vi "InstrumentSelection.vi"(8 "error in (no error)":errorcluster, 9 "Verify GPIB address":bool, 10 "Instrument type":T1(ring), 11 "Instrument name IN":string(combo)) -> (0 "error out":errorcluster, 1 "Instrument name OUT":string, 2 "LCR":refnum<class "LCRControl.lvclass">, 3 "Supply":refnum<class "SupplyControl.lvclass">, 4 "Switching":refnum<class "Switching.lvclass">, 5 "Multimeter":refnum<class "MultimeterControl.lvclass">)   [LabVIEW 2019, in "InstrControl.lvclass"]
uses:
  InstrControl.lvclass
  SupplyControl/SupplyControl.lvclass
  C:/Users/probe/Desktop/TRIUMF-Dark-Box/InstrControl/InstrControl.lvclass
  LCRControl/LCRControl.lvclass
  MultimeterControl/MultimeterControl.lvclass
  Switching/Switching.lvclass
  SupplyControl/Keithley 2410/KE2410.lvclass
  C:/Users/probe/Desktop/TRIUMF-Dark-Box/InstrControl/SupplyControl/SupplyControl.lvclass
  SupplyControl/Keithley 6517/KE6517.lvclass
  SupplyControl/Keithley 487/KE487.lvclass
  SupplyControl/Keithley 236 & 237/KE236.lvclass
  LCRControl/WK6440B/WK6440B.lvclass
  C:/Users/probe/Desktop/TRIUMF-Dark-Box/InstrControl/LCRControl/LCRControl.lvclass
  LCRControl/WK6425/WK6425.lvclass
  MultimeterControl/Keithley 2000/KE2000.lvclass
  C:/Users/probe/Desktop/TRIUMF-Dark-Box/InstrControl/MultimeterControl/MultimeterControl.lvclass
  Switching/Pickering/Pickering.lvclass
  C:/Users/probe/Desktop/TRIUMF-Dark-Box/InstrControl/Switching/Switching.lvclass
  InstrumentSetup.vi
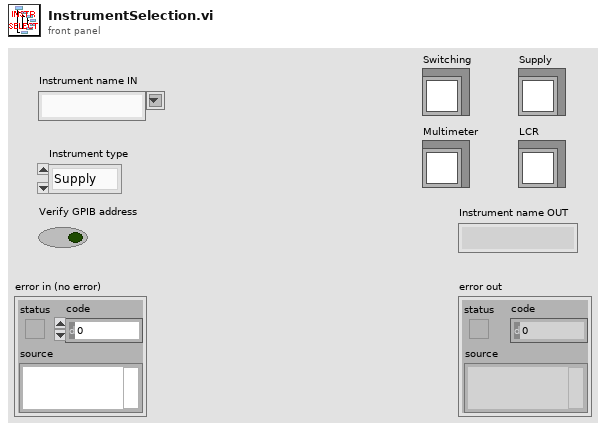
[diagram p1: front panel]
types:
  T1 = enum16{"Supply", "LCR", "Multimeter", "Switching"}
  T2 = cluster{"KE 2410":cluster{"Instrument name":string, "GPIB address":string, "Instrument type":u16}, "KE 6517":cluster{"Instrument name":string, "GPIB address":string, "Instrument type":u16}, "KE 487":cluster{"Instrument name":string, "GPIB address":string, "Instrument type":u16}, "KE 236":cluster{"Instrument name":string, "GPIB address":string, "Instrument type":u16}, "KE 487_2":cluster{"Instrument name":string, "GPIB address":string, "Instrument type":u16}, "WK 6440B":cluster{"Instrument name":string, "GPIB address":string, "Instrument type":u16}, "WK 6425":cluster{"Instrument name":string, "GPIB address":string, "Instrument type":u16}, "Pickering Matrix":cluster{"Instrument name":string, "GPIB address":string, "Instrument type":u16}, "KE 2000":cluster{"Instrument name":string, "GPIB address":string, "Instrument type":u16}, "KE3706A Switching":cluster{"Instrument name":string, "GPIB address":string, "Instrument type":u16}}
  T3 = cluster{"Current Limit":sgl, "KE2410":refnum<class "KE2410.lvclass">}
  T4 = cluster{"Current Limit":u16, "KE6517":refnum<class "KE6517.lvclass">}
  T5 = cluster{"Compliance":u16, "Range:":u16, "KE487":refnum<class "KE487.lvclass">}
  T6 = cluster{"current \ncompliance level":dbl, "compliance/\nmeasurement range (auto:0)":u16, "KE236":refnum<class "KE236.lvclass">}
  T7 = cluster{"RC Configuration":u16, "AC amplitude [V]":dbl, "AC frequency [Hz]":i32, "WK6440B":refnum<class "WK6440B.lvclass">}
  T8 = cluster{"RC Configuration":u16, "AC amplitude [V]":dbl, "AC frequency [Hz]":i32, "WK6425":refnum<class "WK6425.lvclass">}
  T9 = cluster{"Range":u16, "Range Value":dbl, "Function":u16, "KE2000":refnum<class "KE2000.lvclass">}
  T10 = cluster{"Matrix address":string, "Mux1 address":string, "Mux2 address":string, "Matrix used?":bool, "Pickering":refnum<class "Pickering.lvclass">, "Matrix X Channels":cluster{"Bias Supply / SMU LO":i32, "Bias Supply / SMU HI":i32, "CV Box LO":i32, "CV Box HI":i32, "CV Box LO IN":i32, "CV Box HI IN":i32, "Volt meter LO":i32, "Volt meter HI":i32, "Mux1 C1":i32, "Mux1 C2":i32, "Mux2 C1":i32, "Mux2 C2":i32}}
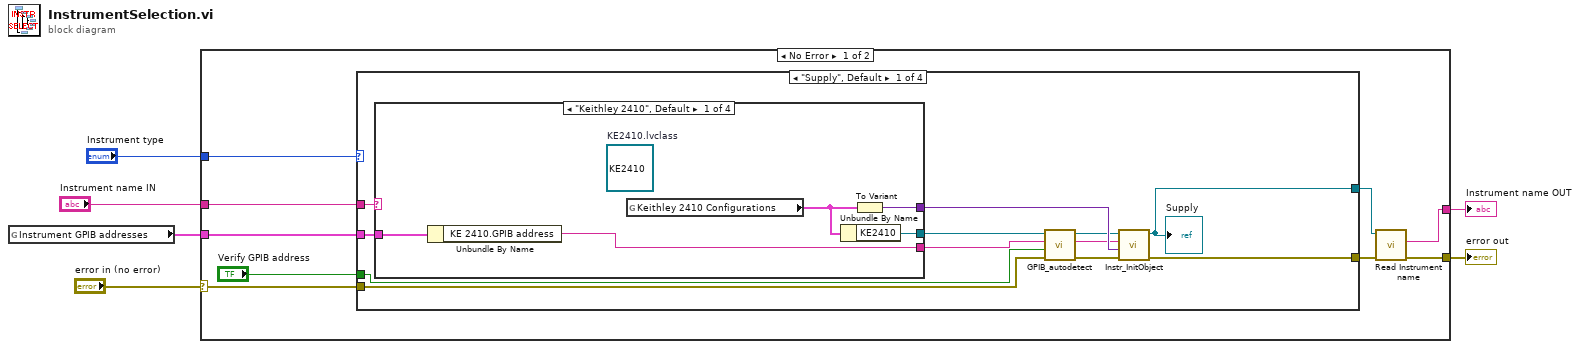
[diagram p0: block diagram]
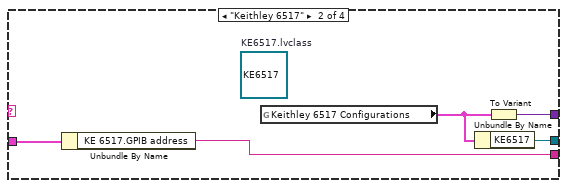
[diagram p2: hidden frame]
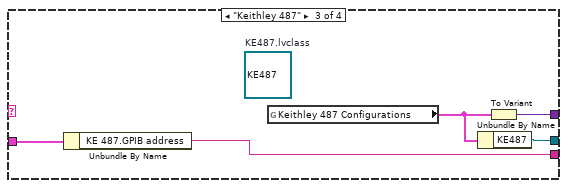
[diagram p3: hidden frame]
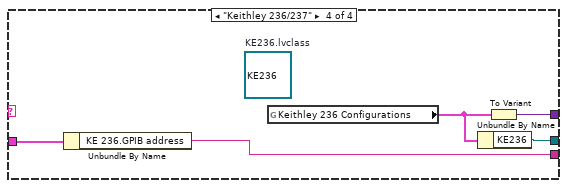
[diagram p4: hidden frame]
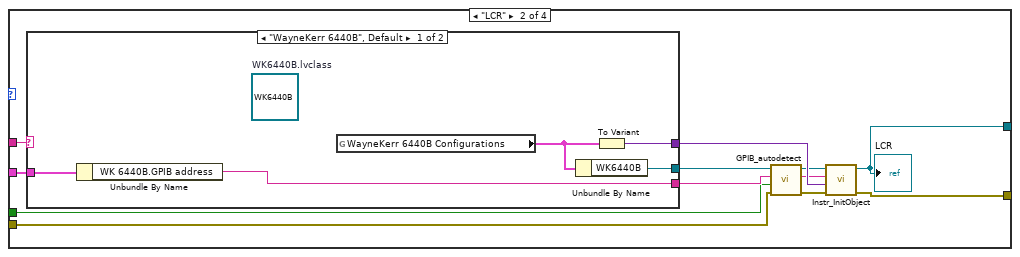
[diagram p5: hidden frame]
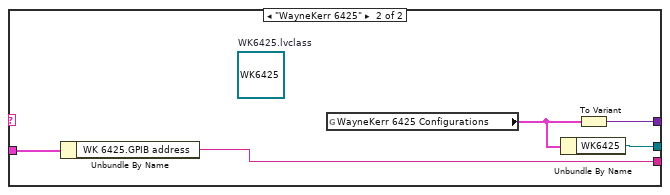
[diagram p6: hidden frame]
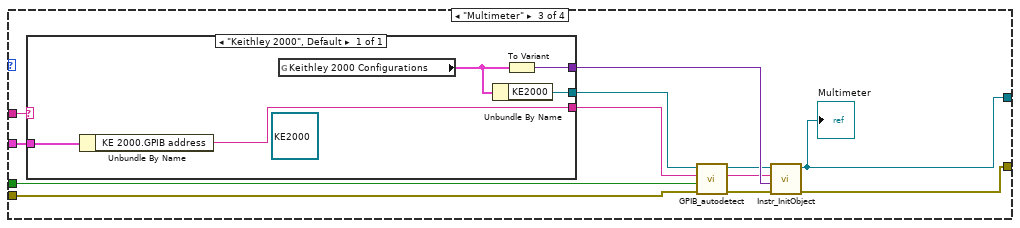
[diagram p7: hidden frame]
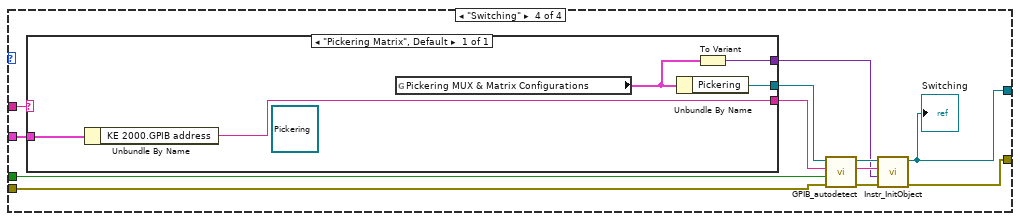
[diagram p8: hidden frame]
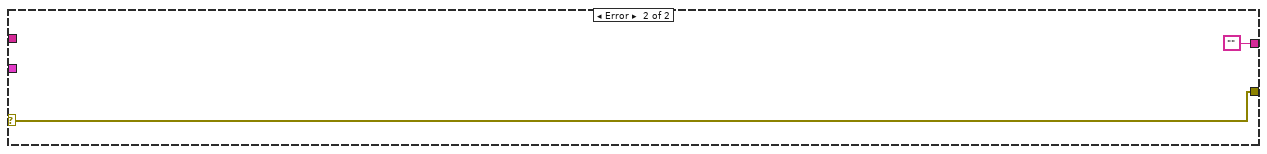
[diagram p9: hidden frame]
diagram:
  n1 = global read "InstrumentSetup.vi" "Instrument GPIB addresses"() -> (w1:T2)
  n2 = case shown="No Error" "error in (no error)" {
    selector: "error in (no error)" -> [w13 w105]
    tunnel: [w14 w105] -> w5
    tunnel: [w15 ""] -> w4
    tunnel: "Instrument type" -> [w10 _]
    tunnel: "Instrument name IN" -> [w9 _]
    tunnel: w1 -> [w8 _]
    frame No Error {
      n3 = case shown="\"Supply\", Default" w10 {
        tunnel: w9 -> [w27 w59 w81 w89]
        tunnel: [w26 w57 w79 w97] -> w12
        tunnel: w13 -> [w18 w54 w71 w91]
        tunnel: [w25 w58 w80 w98] -> w11
        tunnel: w8 -> [w24 w56 w78 w95]
        tunnel: "Verify GPIB address" -> [w17 w48 w76 w90]
        frame "Supply", Default {
          n4 = case shown="\"Keithley 2410\", Default" w27 {
            tunnel: [w29 w33 w38 w43] -> w20
            tunnel: w24 -> [w32 w37 w42 w47]
            tunnel: [w31 w36 w41 w46] -> w22
            tunnel: [w30 w35 w40 w45] -> w23
            frame "Keithley 2410", Default {
              (unwired) refnum<class "KE2410.lvclass"> refnum  # KE2410.lvclass
              n5 = Unbundle By Name(w32) -> ("KE 2410.GPIB address"=w31:string)
              n6 = global read "InstrumentSetup.vi" "Keithley 2410 Configurations"() -> (w28:T3)
              n7 = Unbundle By Name(w28) -> ("KE2410"=w29:refnum<class "KE2410.lvclass">)
              n8 = To Variant(anything=w28) -> (Variant=w30:variant)
            }
            frame "Keithley 6517" {
              (unwired) refnum<class "KE6517.lvclass"> refnum  # KE6517.lvclass
              n9 = Unbundle By Name(w37) -> ("KE 6517.GPIB address"=w36:string)
              n10 = global read "InstrumentSetup.vi" "Keithley 6517 Configurations"() -> (w34:T4)
              n11 = Unbundle By Name(w34) -> ("KE6517"=w33:refnum<class "KE6517.lvclass">)
              n12 = To Variant(anything=w34) -> (Variant=w35:variant)
            }
            frame "Keithley 487" {
              (unwired) refnum<class "KE487.lvclass"> refnum  # KE487.lvclass
              n13 = Unbundle By Name(w42) -> ("KE 487.GPIB address"=w41:string)
              n14 = global read "InstrumentSetup.vi" "Keithley 487 Configurations"() -> (w39:T5)
              n15 = Unbundle By Name(w39) -> ("KE487"=w38:refnum<class "KE487.lvclass">)
              n16 = To Variant(anything=w39) -> (Variant=w40:variant)
            }
            frame "Keithley 236/237" {
              (unwired) refnum<class "KE236.lvclass"> refnum  # KE236.lvclass
              n17 = Unbundle By Name(w47) -> ("KE 236.GPIB address"=w46:string)
              n18 = global read "InstrumentSetup.vi" "Keithley 236 Configurations"() -> (w44:T6)
              n19 = Unbundle By Name(w44) -> ("KE236"=w43:refnum<class "KE236.lvclass">)
              n20 = To Variant(anything=w44) -> (Variant=w45:variant)
            }
          }
          n21 = call-dynamic "GPIB_autodetect.vi"("error in (no error)"=w18, "Verify GPIB address"=w17, "Instrument GPIB address in"=w22, "InstrControl in"=w20) -> ("error out"=w16:errorcluster, "Instrument GPIB address"=w21:string, "InstrControl out"=w19:refnum<class "SupplyControl.lvclass">)  [unwired: 5 in]
          n22 = call-dynamic "Instr_InitObject.vi"("error in (no error)"=w16, "Instrument Configuration"=w23, "GPIB address"=w21, "SupplyControl in"=w19) -> ("error out"=w25:errorcluster, "SupplyControl out"=w26:refnum<class "SupplyControl.lvclass">)  [unwired: 6 in]
          "Supply" <- w26
        }
        frame "LCR" {
          n23 = case shown="\"WayneKerr 6440B\", Default" w59 {
            tunnel: [w60 w65] -> w50
            tunnel: w56 -> [w64 w69]
            tunnel: [w63 w68] -> w52
            tunnel: [w62 w67] -> w55
            frame "WayneKerr 6440B", Default {
              (unwired) refnum<class "WK6440B.lvclass"> refnum  # WK6440B.lvclass
              n24 = Unbundle By Name(w64) -> ("WK 6440B.GPIB address"=w63:string)
              n25 = global read "InstrumentSetup.vi" "WayneKerr 6440B Configurations"() -> (w61:T7)
              n26 = Unbundle By Name(w61) -> ("WK6440B"=w60:refnum<class "WK6440B.lvclass">)
              n27 = To Variant(anything=w61) -> (Variant=w62:variant)
            }
            frame "WayneKerr 6425" {
              (unwired) refnum<class "WK6425.lvclass"> refnum  # WK6425.lvclass
              n28 = Unbundle By Name(w69) -> ("WK 6425.GPIB address"=w68:string)
              n29 = global read "InstrumentSetup.vi" "WayneKerr 6425 Configurations"() -> (w66:T8)
              n30 = Unbundle By Name(w66) -> ("WK6425"=w65:refnum<class "WK6425.lvclass">)
              n31 = To Variant(anything=w66) -> (Variant=w67:variant)
            }
          }
          n32 = call-dynamic "GPIB_autodetect.vi"("error in (no error)"=w54, "Verify GPIB address"=w48, "Instrument GPIB address in"=w52, "InstrControl in"=w50) -> ("error out"=w53:errorcluster, "Instrument GPIB address"=w51:string, "InstrControl out"=w49:refnum<class "LCRControl.lvclass">)  [unwired: 5 in]
          n33 = call-dynamic "Instr_InitObject.vi"("error in (no error)"=w53, "Instrument Configuration"=w55, "GPIB Address"=w51, "LCRControl in"=w49) -> ("error out"=w58:errorcluster, "LCRControl out"=w57:refnum<class "LCRControl.lvclass">)  [unwired: 6 in]
          "LCR" <- w57
        }
        frame "Multimeter" {
          n34 = case shown="\"Keithley 2000\", Default" w81 {
            tunnel: [w82] -> w72
            tunnel: w78 -> [w86]
            tunnel: [w85] -> w75
            tunnel: [w84] -> w77
            frame "Keithley 2000", Default {
              (unwired) refnum<class "KE2000.lvclass"> refnum ("KE2000.lvclass")
              n35 = Unbundle By Name(w86) -> ("KE 2000.GPIB address"=w85:string)
              n36 = global read "InstrumentSetup.vi" "Keithley 2000 Configurations"() -> (w83:T9)
              n37 = Unbundle By Name(w83) -> ("KE2000"=w82:refnum<class "KE2000.lvclass">)
              n38 = To Variant(anything=w83) -> (Variant=w84:variant)
            }
          }
          n39 = call-dynamic "GPIB_autodetect.vi"("error in (no error)"=w71, "Verify GPIB address"=w76, "Instrument GPIB address in"=w75, "InstrControl in"=w72) -> ("error out"=w70:errorcluster, "Instrument GPIB address"=w74:string, "InstrControl out"=w73:refnum<class "KE2000.lvclass">)  [unwired: 5 in]
          n40 = call-dynamic "Instr_InitObject.vi"("error in (no error)"=w70, "Instrument Configuration"=w77, "GPIB Address"=w74, "KE2000 in"=w73) -> ("error out"=w80:errorcluster, "KE2000 out"=w79:refnum<class "KE2000.lvclass">)  [unwired: 6 in]
          "Multimeter" <- w79
        }
        frame "Switching" {
          n41 = case shown="\"Pickering Matrix\", Default" w89 {
            tunnel: w95 -> [w103]
            tunnel: [w102] -> w94
            tunnel: [w100] -> w88
            tunnel: [w99] -> w87
            frame "Pickering Matrix", Default {
              (unwired) refnum<class "Pickering.lvclass"> refnum ("Pickering")
              n42 = Unbundle By Name(w103) -> ("KE 2000.GPIB address"=w102:string)
              n43 = global read "InstrumentSetup.vi" "Pickering MUX & Matrix Configurations"() -> (w101:T10)
              n44 = Unbundle By Name(w101) -> ("Pickering"=w99:refnum<class "Pickering.lvclass">)
              n45 = To Variant(anything=w101) -> (Variant=w100:variant)
            }
          }
          n46 = call-dynamic "GPIB_autodetect.vi"("error in (no error)"=w91, "Verify GPIB address"=w90, "Instrument GPIB address in"=w94, "InstrControl in"=w87) -> ("error out"=w93:errorcluster, "Instrument GPIB address"=w92:string, "InstrControl out"=w96:refnum<class "Pickering.lvclass">)  [unwired: 5 in]
          n47 = call-dynamic "Instr_InitObject.vi"("error in (no error)"=w93, "Instrument Configuration"=w88, "GPIB Address"=w92, "Pickering in"=w96) -> ("error out"=w98:errorcluster, "Pickering out"=w97:refnum<class "Pickering.lvclass">)  [unwired: 6 in]
          "Switching" <- w97
        }
      }
      n48 = call-dynamic "Read Instrument name.vi"("error in (no error)"=w11, "InstControl in"=w12) -> ("error out"=w14:errorcluster, "Instrument name"=w15:string)  [unwired: 7 in, 1 out]
    }
    frame Error {
    }
  }
  "error out" <- w5
  "Instrument name OUT" <- w4
